vi "Create Table Query.vi"(8 "error in (no error)":errorcluster, 9 "Column Definition Strings":string[](array[string]), 10 "Table Name":string, 11 "PostgreSQL in":refnum<class "PostgreSQL.lvclass">) -> (0 "error out":errorcluster, 1 "Create Table Query":string, 3 "PostgreSQL out":refnum<class "PostgreSQL.lvclass">)   [LabVIEW 2018, in "Database.lvlib" / "PostgreSQL.lvclass"]
uses:
  PostgreSQL.lvclass
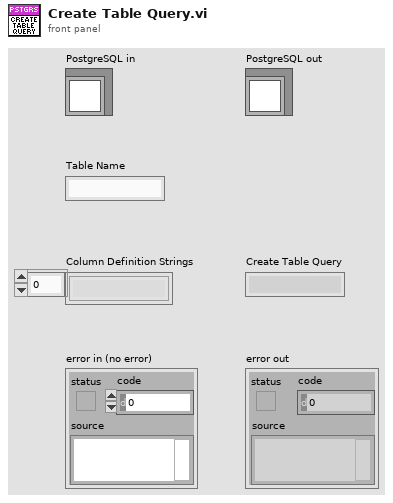
[diagram p1: front panel]
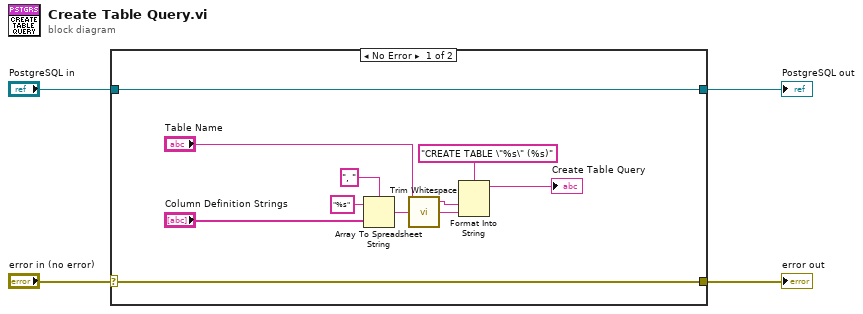
[diagram p0: block diagram]
diagram:
  n1 = case shown="No Error" "error in (no error)" {
    selector: "error in (no error)" -> [w13 w15]
    tunnel: "PostgreSQL in" -> [w14 w16]
    tunnel: [w14 w16] -> w3
    tunnel: [w13 w15] -> w1
    frame No Error {
      n2 = Array To Spreadsheet String(delimiter (Tab)=", ", array="Column Definition Strings", 3:"%s" ("format string")) -> (spreadsheet string=w11:string)
      n3 = call <vilib>:"Trim Whitespace.vi"("string"=w11) -> ("trimmed string"=w8:string)  [unwired: 1 in]
      n4 = Format Into String(format string="CREATE TABLE \"%s\" (%s)", "Table Name", w8) -> (resulting string=→"Create Table Query":string)  [unwired: 2 in, 1 out]
    }
    frame Error {
    }
  }
  "error out" <- w1
  "PostgreSQL out" <- w3
